vi "Module Type.vi"(11 "ValveControlModule in":refnum<class "ValveControlModule.lvclass">) -> (2 "Module Type":string)   [LabVIEW 2020, in "VolatusControl.lvlib" / "ValveControlModule.lvclass"]
uses:
  ValveControlModule.lvclass
  ValveControlModule.lvclass/ValveControlModule.ctl
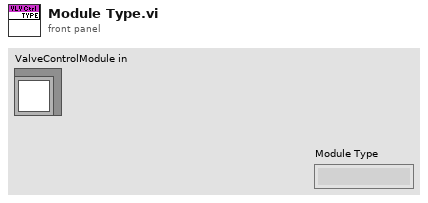
[diagram p1: front panel]
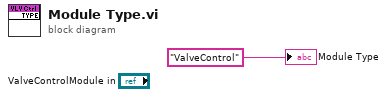
[diagram p0: block diagram]
diagram:
  "Module Type" <- "ValveControl" ("Module Type")
